vi "gfitsio-read-key-string.vi"(7 "keyname":string, 8 "error in (no error)":errorcluster, 9 "default value":string, 11 "gfits refnum":T1) -> (0 "error out":errorcluster, 1 "comment":string, 2 "value":string, 3 "dup gfits refnum":T1)   [LabVIEW 2015, in "gfitsio.lvlib"]
doc: "Return the specified keyword. <B>default value</B> specifies the desired returned data type of the keyword value. Data type conversion will be performed for numeric values if the keyword value does not have the same data type. If the keyword does not exist or an error occurs <B>value</B> will be equal to <B>default value</B>."
uses:
  gfitsio.lvlib
  gfitsio-refnum.ctl
  cfitsio-datatypes.ctl
  gfitsio_32Bit/gfitsio.dll
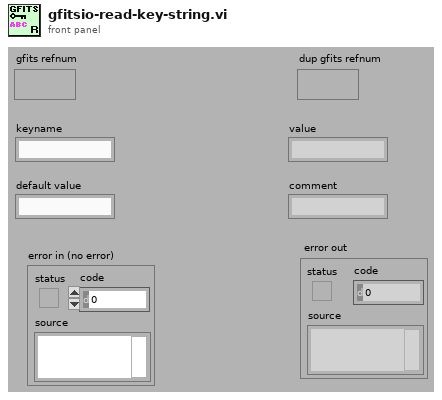
[diagram p1: front panel]
types:
  T1 = typedef "gfitsio.lvlib/gfitsio-refnum.ctl" = refnum<k1>
  T2 = typedef "gfitsio.lvlib/cfitsio-datatypes.ctl" = i32
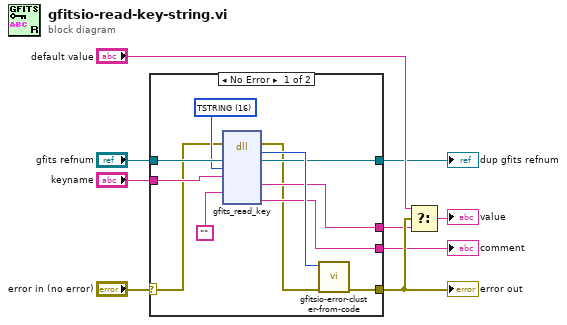
[diagram p0: block diagram]
diagram:
  n1 = case shown="No Error" "error in (no error)" {
    selector: "error in (no error)" -> [w11 w22]
    tunnel: [w19 w22] -> w4
    tunnel: "gfits refnum" -> [w17 w21]
    tunnel: [w18 w21] -> w1
    tunnel: "keyname" -> [w15 _]
    tunnel: [w14 _] -> w2
    tunnel: [w13 _] -> w3
    frame No Error {
      w16 = T2 16 items=["TBIT"=1, "TBYTE  (U8)"=11, "TSBYTE  (I8)"=12, "TLOGICAL"=14, "TSTRING"=16, "TUSHORT  (U16)"=20, "TSHORT  (I16)"=21, "TUINT"=31, "TULONG  (U32)"=40, "TLONG  (I32)"=41, "TFLOAT  (SGL)"=42, "TLONGLONG  (I64)"=81, "TDOUBLE"=82, "TCOMPLEX  (CSG)"=83, "TDOUBLECOMPLEX  (CDB)"=163] ("cfitsio datatype")
      n2 = dll-call lib="C:/GSCS 2.0/GSCS/Systems/SIcamera_Control/Quick_Look/gfitsio_32Bit/gfitsio.dll" fn="gfits_read_key"(error in=w11, "refnum"=w17, "datatype"=w16, "keyname"=w15, "units"="") -> (error out=w10:errorcluster, "return type"=w20:i32, "refnum"=w18:T1, "value"=w14:string, "comment"=w13:string)  [unwired: 4 in, 4 out]
      n3 = call "gfitsio-error-cluster-from-code.vi"("error in (no error)"=w10, "error code"=w20) -> ("error out"=w19:errorcluster)  [unwired: 9 out]
    }
    frame Error {
    }
  }
  "error out" <- w4
  "dup gfits refnum" <- w1
  "comment" <- w3
  n4 = Select(t="default value", s=w4, f=w2) -> (s? t:f=→"value":string)
